vi "LcXSDSOAcqData.vi"() -> ()   [LabVIEW 2022 SP3]
panel:
  in  "Case Constant\n(See Context Help) 2":bool
  in  "Case Constant\n(See Context Help)":bool
  out "Att (dB)":dbl[](array[numeric]) format="%.2f"
  in  "Channel to pull":i32=1
  in  "Channels to Acq":i32=1
  in  "OK Button":bool=TRUE
  in  "input imp (Mohms)":dbl(ring)=50.0 items=["50.0 ohms"=50.0, "75.0 ohms"=75.0, "1.0 mega ohm"=1000000.0]
  in  "instrument handle out":refnum<k15>
  in  "Num of Sequences":i32=10
  in  "Seq Num to pull":i32=1
  in  "Delay (micsec)":dbl format="%.1f"
  in  "Sampling Rate":u16(ring)=5
  in  "rf points":i32=2000
  in  "trigger level (volts)":dbl=0.1 format="%.2f"
  in  "trigger source":string(combo)="VAL_EXTERNAL"
  in  "trigger slope":i32(slide)=1
  in  "trigger holdoff (micsec)":dbl format="%.2f"
  out "Actual Samp Rate (MHz)":dbl
  out "Waveform Graph":cluster{i32, dbl, "Data":i16[]}(graph)
  out "actual points":i32
  out "error out":errorcluster
  in  "resource name":string="VICP::LCRY0602P10739"
  # "Use, for example, the scope output signal connected to channel C1"
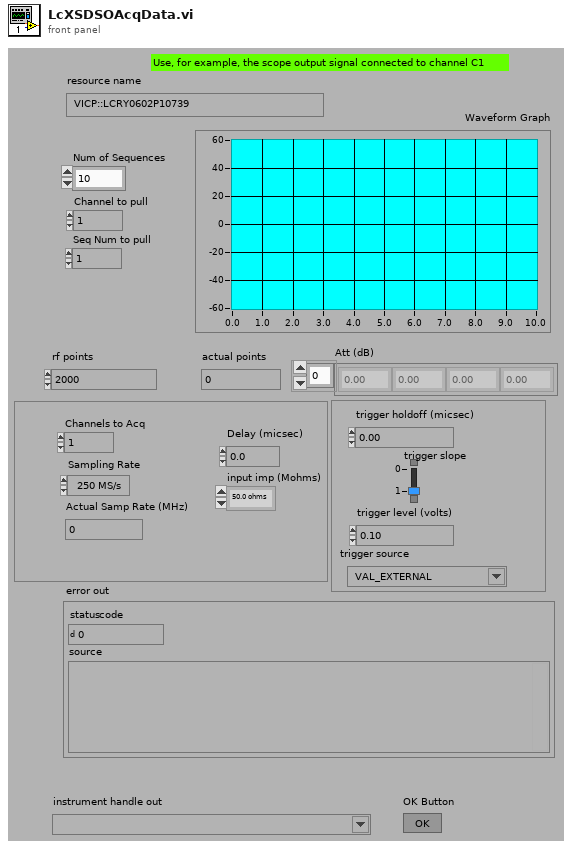
[diagram p1: front panel]
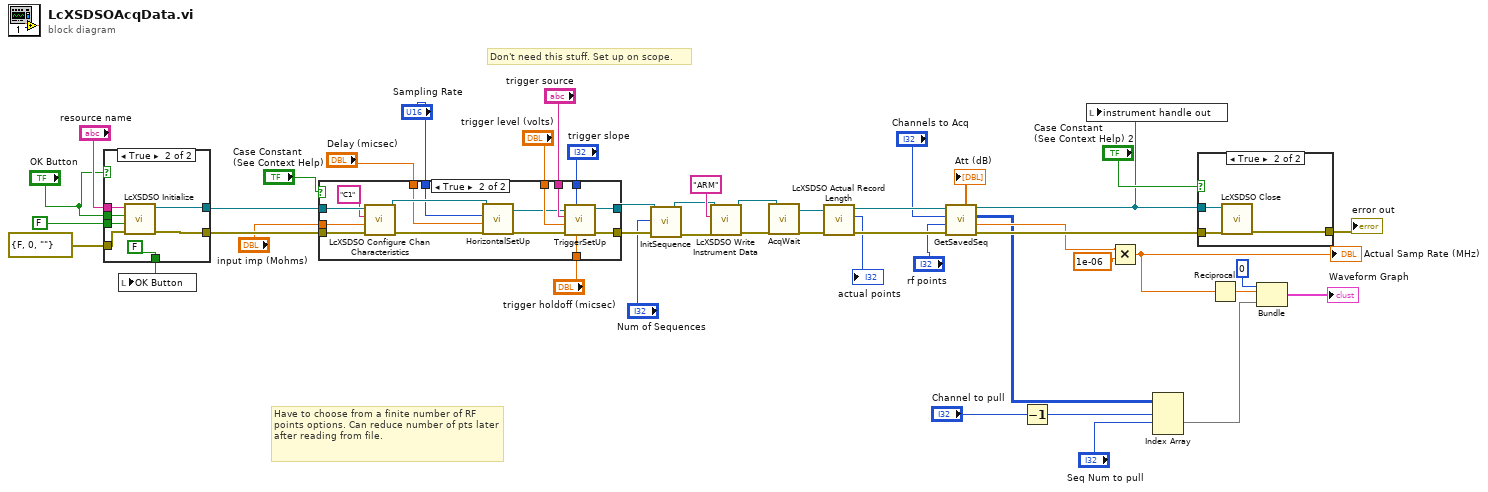
[diagram p0: block diagram]
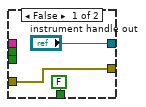
[diagram p4: hidden frame]
diagram:
  # "Don't need this stuff. Set up on scope."
  # "Have to choose from a finite number of RF points options. Can reduce number of pts later after reading from file."
  n1 = case shown="True" "OK Button" {
    tunnel: errorcluster {"status"=FALSE, "code"=0, "source"=""} ("error in (no error)") -> [w49 w56]
    tunnel: "resource name" -> [_ w55]
    tunnel: "OK Button" -> [_ w54]
    tunnel: FALSE ("reset device") -> [_ w53]
    tunnel: [w49 w52] -> w36
    tunnel: ["instrument handle out" w51] -> w20
    tunnel: [FALSE FALSE] -> w23
    frame False {
    }
    frame True {
      n2 = call "LcXSDSO Initialize.vi"("error in (no error)"=w56, "reset device"=w53, "id query"=w54, "resource name"=w55) -> ("error out"=w52:errorcluster, "instrument handle out"=w51:refnum<k15>)  [unwired: 6 in]
    }
  }
  n3 = local write "OK Button"(w23) -> ()
  n4 = case shown="True" "Case Constant\n(See Context Help)" {
    tunnel: "trigger holdoff (micsec)" -> [_ w74]
    tunnel: "trigger slope" -> [_ w73]
    tunnel: "trigger source" -> [_ w72]
    tunnel: "trigger level (volts)" -> [_ w71]
    tunnel: "Sampling Rate" -> [_ w60]
    tunnel: "Delay (micsec)" -> [_ w59]
    tunnel: w36 -> [w58 w70]
    tunnel: "input imp (Mohms)" -> [_ w69]
    tunnel: w20 -> [w57 w68]
    tunnel: [w58 w66] -> w6
    tunnel: [w57 w65] -> w5
    frame False {
    }
    frame True {
      n5 = call "LcXSDSO Configure Chan Characteristics.vi"("error in (no error)"=w70, "input impedance (ohms)"=w69, "channel name"="C1", "instrument handle"=w68) -> ("error out"=w61:errorcluster, "instrument handle out"=w62:refnum<k15>)  [unwired: 6 in]
      n6 = call "HorizontalSetUp.vi"("ActXDSO In"=w62, "Sampling Rate"=w60, "Delay (micsec)"=w59, "error in"=w61) -> ("ActXDSO Out"=w64:refnum<k7>, "error out"=w63:errorcluster)  [unwired: 1 in]
      n7 = call "TriggerSetUp.vi"("trigger holdoff (micsec)"=w74, "trigger slope"=w73, "errorin"=w63, "trigger level (volts)"=w71, "trigger source"=w72, "instrument handle in"=w64) -> ("error out"=w66:errorcluster, "inst handle out"=w65:refnum<k15>)
    }
  }
  n8 = call "InitSequence.vi"("ActXDSO In"=w5, "Num of Sequences"="Num of Sequences", "error in (no error)"=w6) -> ("ActXDSO Out"=w8:refnum<k7>, "error out"=w7:errorcluster)  [unwired: 4 in]
  n9 = call "LcXSDSO Write Instrument Data.vi"("error in (no error)"=w7, "write buffer"="ARM", "instrument handle"=w8) -> ("error out"=w26:errorcluster, "instrument handle out"=w27:refnum<k15>)  [unwired: 7 in]
  n10 = call "AcqWait.vi"("error in"=w26, "ActXDSO In"=w27) -> ("error out"=w35:errorcluster, "ActXDSO Out"=w34:refnum<k7>)
  n11 = call "LcXSDSO Actual Record Length.vi"("error in (no error)"=w35, "instrument handle"=w34) -> ("error out"=w33:errorcluster, "actual  record length"=→"actual points":i32, "instrument handle out"=w32:refnum<k15>)  [unwired: 7 in]
  n12 = call "GetSavedSeq.vi"("error in (no error)"=w33, "RF Points"="rf points", "Channels to Acq"="Channels to Acq", "instrument handle"=w32) -> ("error out"=w37:errorcluster, "Samp Rate"=w29:sgl, "Data"=w14:i16[][][], "instrument handle out"=w19:refnum<k15>, "Att (dB)"=→"Att (dB)":dbl[])  [unwired: 3 in]
  n13 = Decrement(x="Channel to pull") -> (x-1=w10:i32)
  n14 = local write "instrument handle out"(w19) -> ()
  n15 = Multiply(x=w29, y=1e-06) -> (x*y=w28:dbl)
  "Actual Samp Rate (MHz)" <- w28
  n16 = Index Array(array=w14, index (dim 0)=w10, index (dim 1)="Seq Num to pull") -> (element=w16:i16[])  [unwired: 1 in]
  n17 = case shown="True" "Case Constant\n(See Context Help) 2" {
    tunnel: [w75 w78] -> w43
    tunnel: w19 -> [_ w77]
    tunnel: w37 -> [w75 w76]
    frame False {
    }
    frame True {
      n18 = call "LcXSDSO Close.vi"("error in (no error)"=w76, "instrument handle"=w77) -> ("error out"=w78:errorcluster)  [unwired: 9 in]
    }
  }
  "error out" <- w43
  n19 = Reciprocal(x=w28) -> (1/x=w30:dbl)
  n20 = Bundle "Bundle"(0, w30, "Data"=w16) -> (→"Waveform Graph":cluster{i32, dbl, "Data":i16[]})  [unwired: 1 in]
